vi "ROI Inicial.vi"(0 "Image in":T1, 1 "error in (no error)":errorcluster) -> (2 "Image out":T1, 3 "ROI Descriptor":T2 {"Contours"."Type" items=["No Selection", "Point", "Line", "Rectangle", "Oval", "Polygon", "Freehand Region", "Annulus", "Unused2", "Unused3", "Broken Line", "Freehand Line", "Rotated Rectangle"]}, 4 "error out":errorcluster)   [LabVIEW 2020]
uses:
  <vilib>/vision/Image Controls.llb/IMAQ Image.ctl
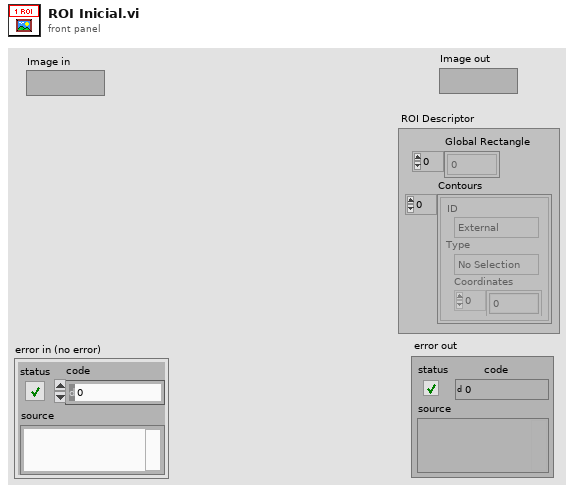
[diagram p1: front panel]
types:
  T1 = typedef "IMAQ Image.ctl" = refnum<image>
  T2 = typedef "ROI Descriptor" = cluster{"Global Rectangle":i32[], "Contours":cluster{"ID":enum32{"External", "Internal"}, "Type":u32, "Coordinates":i32[]}[]}
  T3 = typedef "IMAQ Rectangle" = cluster{"Left":i32, "Top":i32, "Right":i32, "Bottom":i32, "Rotation":dbl}
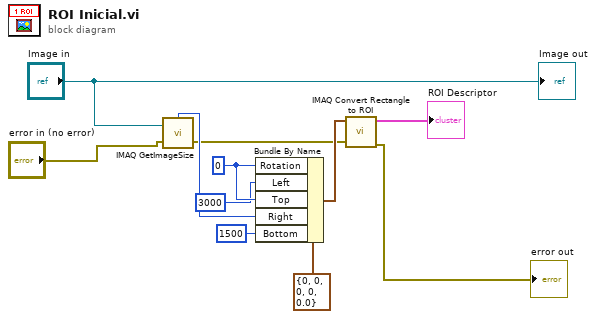
[diagram p0: block diagram]
diagram:
  w11 = 0 ("Left")
  n1 = call "IMAQ GetImageSize"("Image"="Image in", "error in (no error)"="error in (no error)") -> ("X Resolution"=w9:i32, "error out"=w6:errorcluster)  [unwired: 2 in, 1 out]
  n2 = Bundle By Name(cluster=T3 {"Left"=0, "Top"=0, "Right"=0, "Bottom"=0, "Rotation"=0.0} ("Rectangle"), "Rotation"=w11, "Left"=3000, "Top"=w11, "Right"=w9, "Bottom"=1500) -> (w8:T3)
  n3 = call "IMAQ Convert Rectangle to ROI"("error in (no error)"=w6, "Rectangle"=w8) -> ("error out"=→"error out":errorcluster, "ROI Descriptor"=→"ROI Descriptor":T2)  [unwired: 7 in]
  "Image out" <- "Image in"
